vi "Get Full Help.vi"(8 "error in (no error)":errorcluster, 11 "Package in":refnum<class "Package.lvclass">) -> (0 "error out":errorcluster, 2 "Full Help":string, 3 "Package out":refnum<class "Package.lvclass">)   [LabVIEW 2020, in "Package.lvlib" / "Package.lvclass"]
uses:
  Package.lvclass
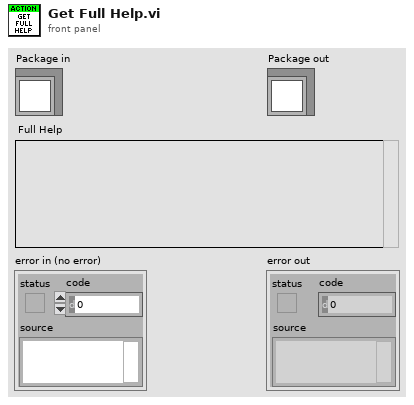
[diagram p1: front panel]
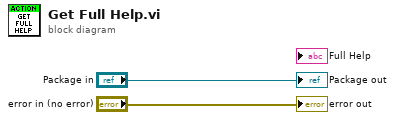
[diagram p0: block diagram]
diagram:
  "error out" <- "error in (no error)"
  "Package out" <- "Package in"
